vi "Is Sleeping.vi"(8 "error in (no error)":errorcluster, 11 "Baby in":refnum<class "Baby.lvclass">) -> (0 "error out":errorcluster, 2 "IsSleeping":bool, 3 "Baby out":refnum<class "Baby.lvclass">)   [LabVIEW 2009, in "Baby.lvclass"]
doc: "Check on baby to see if she's sleeping."
uses:
  Baby.lvclass
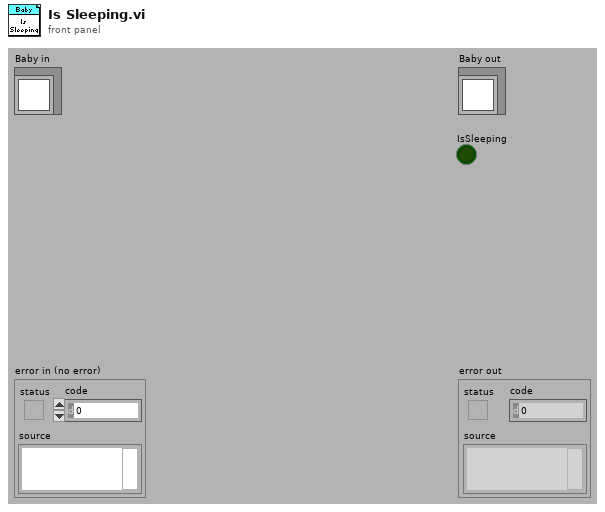
[diagram p1: front panel]
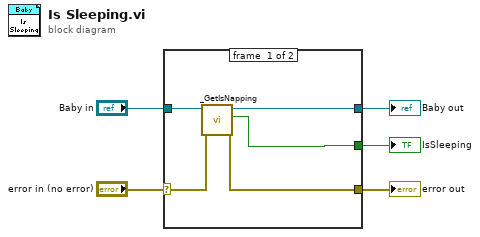
[diagram p0: block diagram]
diagram:
  n1 = case shown="No Error" "error in (no error)" {
    selector: "error in (no error)" -> [w8 w12]
    tunnel: [w7 w12] -> w4
    tunnel: [w9 w11] -> w2
    tunnel: "Baby in" -> [w10 w11]
    tunnel: [w6 _] -> w1
    frame #0 {
      n2 = call "_GetIsNapping.vi"("error in (no error)"=w8, "Baby in"=w10) -> ("error out"=w7:errorcluster, "IsNapping"=w6:bool, "Baby out"=w9:refnum<class "Baby.lvclass">)  [unwired: 7 in]
    }
    frame #1 {
    }
  }
  "error out" <- w4
  "Baby out" <- w2
  "IsSleeping" <- w1
